vi "Set Filter.vi"(8 "error in (no error)":errorcluster, 9 "Filter Value":u8, 11 "Honeywell Compass HMC6343":refnum<class "Honeywell Compass HMC6343.lvclass">) -> (0 "error out":errorcluster, 3 "Honeywell Compass HMC6343 out":refnum<class "Honeywell Compass HMC6343.lvclass">)   [LabVIEW 2019, in "Honeywell Compass HMC6343.lvclass"]
doc: "Changes the filter value. This allows for an Infinite Impulse Response (IIR) filter to be employed on current and previous heading data outputs. Typical values are 0 to 15 with a factory default of zero. The filter is only applied in run mode where a continuous stream of data is present."
uses:
  Honeywell Compass HMC6343.lvclass
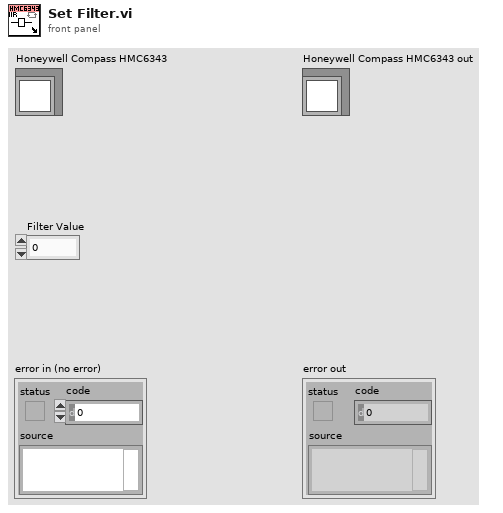
[diagram p1: front panel]
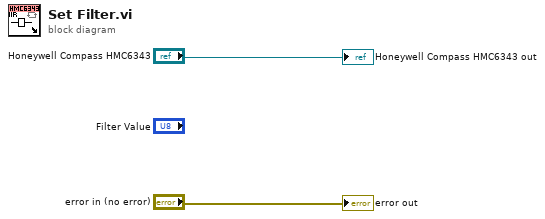
[diagram p0: block diagram]
diagram:
  "error out" <- "error in (no error)"
  "Honeywell Compass HMC6343 out" <- "Honeywell Compass HMC6343"
